vi "LWXPS_TZPVTPulseOutputGet.vi"(0 "XPS Reference IN":refnum<k24>, 7 "TZ group name":string, 11 "LabVIEW error IN":errorcluster) -> (3 "XPS Reference OUT":refnum<k24>, 4 "Returned error code":i32, 6 "Start element number":i32, 8 "End element number":i32, 10 "Time interval":dbl, 14 "LabVIEW error OUT":errorcluster, 15 "XPS Error String":string)   [LabVIEW 2014]
uses:
  D:/XPSQ8_LabView_Library/Development/Source/Dll/Newport.XPS.CommandInterface.dll
  Dll/Newport.XPS.CommandInterface.dll
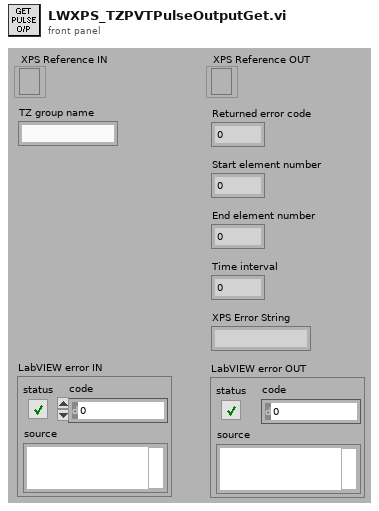
[diagram p1: front panel]
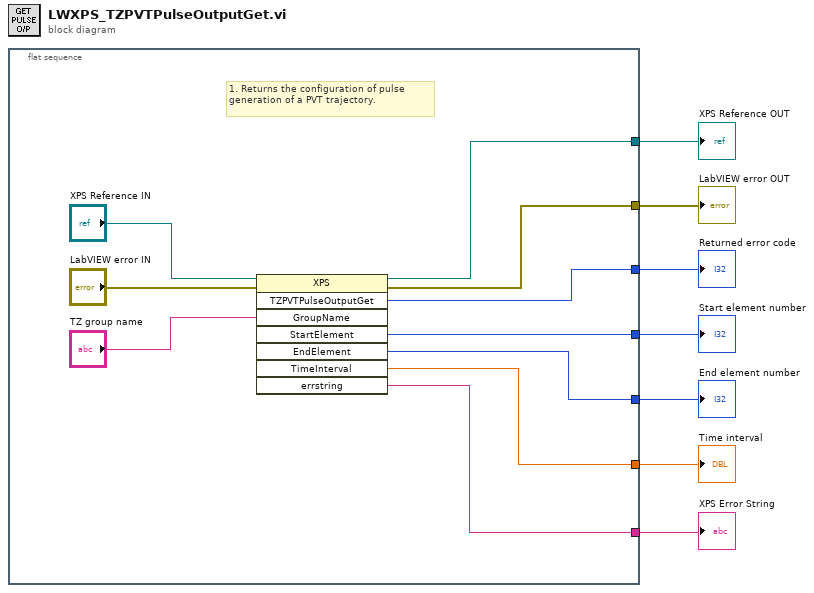
[diagram p0: block diagram]
diagram:
  n1 = flat-sequence {
    tunnel: [w15] -> w7
    tunnel: [w13] -> w6
    tunnel: [w16] -> w5
    tunnel: [w11] -> w3
    tunnel: [w12] -> w2
    tunnel: [w10] -> w1
    tunnel: [w9] -> w4
    frame #0 {
      # "1. Returns the configuration of pulse generation of a PVT trajectory."
      n2 = invoke class="XPS" method="TZPVTPulseOutputGet"(reference="XPS Reference IN", error in="LabVIEW error IN", "GroupName"="TZ group name") -> (reference out=w15:refnum<k24>, error out=w13:errorcluster, "TZPVTPulseOutputGet"=w16:i32, "StartElement"=w11:i32, "EndElement"=w12:i32, "TimeInterval"=w10:dbl, "errstring"=w9:string)  [unwired: 5 in, 1 out]
    }
  }
  "XPS Error String" <- w4
  "XPS Reference OUT" <- w7
  "LabVIEW error OUT" <- w6
  "Returned error code" <- w5
  "Start element number" <- w3
  "End element number" <- w2
  "Time interval" <- w1
